vi "TrajOffset.vi"(4 "OffsetNo":i16, 5 "Offsets":dbl[](array[numeric]), 6 "StartPos":dbl[](array[numeric]), 7 "Repeat number":i16, 8 "error in":errorcluster, 9 "Acc":dbl, 10 "Vel":dbl, 11 "FileName":string) -> (0 "error out":errorcluster)   [LabVIEW 2022 SP3]
uses:
  Global 3.vi
  Newport.XPS.CommandInterface
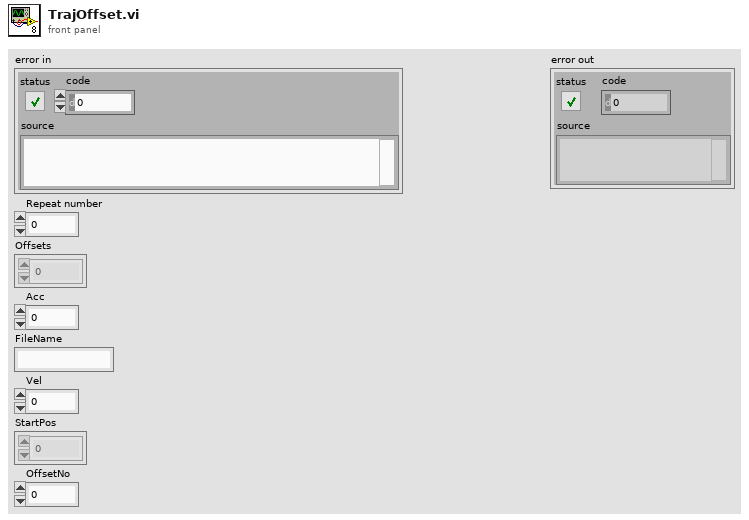
[diagram p1: front panel]
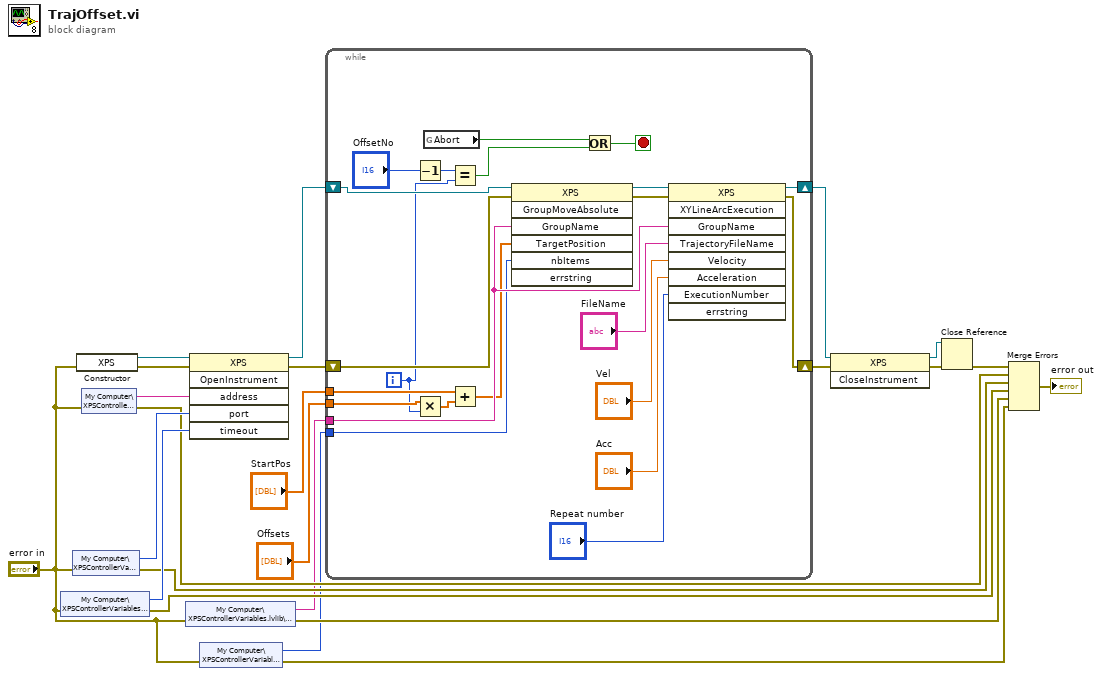
[diagram p0: block diagram]
diagram:
  n1 = shared-variable "My Computer\\XPSControllerVariables.lvlib\\Timeout"(error in="error in") -> (w19:i16, error out=w12:errorcluster)
  n2 = shared-variable "My Computer\\XPSControllerVariables.lvlib\\Port"(error in="error in") -> (w20:i16, error out=w13:errorcluster)
  n3 = constructor class="XPS"(error in="error in") -> (reference out=w23:refnum<k24>, error out=w22:errorcluster)  [unwired: 2 in, 1 out]
  n4 = shared-variable "My Computer\\XPSControllerVariables.lvlib\\IP"(error in="error in") -> (w21:string, error out=w14:errorcluster)
  n5 = shared-variable "My Computer\\XPSControllerVariables.lvlib\\GroupName"(error in="error in") -> (w6:string, error out=w11:errorcluster)
  n6 = invoke class="XPS" method="OpenInstrument"(reference=w23, error in=w22, "address"=w21, "port"=w20, "timeout"=w19) -> (reference out=w8:refnum<k24>, error out=w7:errorcluster)  [unwired: 1 in, 4 out]
  n7 = shared-variable "My Computer\\XPSControllerVariables.lvlib\\nbitem"(error in="error in") -> (w5:i16, error out=w3:errorcluster)
  n8 = while {
    tunnel: w6 -> [w35]
    tunnel: w5 -> [w34]
    shift-right: [w42] -> w18
    shift-left: w8 -> [w39]
    shift-right: [w41] -> w17
    shift-left: w7 -> [w38]
    tunnel: "StartPos" -> [w32]
    tunnel: "Offsets" -> [w31]
    i -> [w27]
    stop <- w26 stop-if-true
    n9 = Decrement(x="OffsetNo") -> (x-1=w28:i16)
    n10 = Multiply(x=w31, y=w27) -> (x*y=w30:dbl[])
    n11 = global read "Global 3.vi" "Abort"() -> (w24:bool)
    n12 = Equal?(x=w28, y=w27) -> (x = y?=w25:bool)
    n13 = Add(x=w32, y=w30) -> (x+y=w33:dbl[])
    n14 = invoke class="XPS" method="GroupMoveAbsolute"(reference=w39, error in=w38, "GroupName"=w35, "TargetPosition"=w33, "nbItems"=w34) -> (reference out=w37:refnum<k24>, error out=w36:errorcluster)  [unwired: 2 in, 5 out]
    n15 = Or(x=w24, y=w25) -> (x .or. y?=w26:bool)
    n16 = invoke class="XPS" method="XYLineArcExecution"(reference=w37, error in=w36, "GroupName"=w35, "TrajectoryFileName"="FileName", "Velocity"="Vel", "Acceleration"="Acc", "ExecutionNumber"="Repeat number") -> (reference out=w42:refnum<k24>, error out=w41:errorcluster)  [unwired: 2 in, 7 out]
  }
  n17 = invoke class="XPS" method="CloseInstrument"(reference=w18, error in=w17) -> (reference out=w16:refnum<k24>, error out=w15:errorcluster)  [unwired: 1 in, 1 out]
  n18 = Close Reference(reference=w16, error in (no error)=w15) -> (error out=w10:errorcluster)
  n19 = Merge Errors(w10, w14, w13, w12, w11, w3) -> (→"error out":errorcluster)
